vi "PID.vi"() -> ()   [LabVIEW 2016]
uses:
  <vilib>/addons/control/pid/autopid.llb/PID autotuning parameters (adv).ctl
  <vilib>/Analysis/baseanly.llb/Mean (DBL).vi
  <userlib>/Fluigent/Fluigent MFCS/FluigentMFCS_Full.llb/MFCS_EZ Detect.vi
  <userlib>/Fluigent/Fluigent MFCS/FluigentMFCS_Full.llb/MFCS_EZ Initialization.vi
  <userlib>/Fluigent/Fluigent MFCS/FluigentMFCS_Full.llb/MFCS_EZ Read All Channels Pressure.vi
  <userlib>/Fluigent/Fluigent MFCS/FluigentMFCS_Full.llb/MFCS_EZ Write Channel Pressure.vi
  <vilib>/addons/control/pid/NI_PID_autopid.lvlib
  <vilib>/Analysis/NI_AALBase.lvlib
  <vilib>/addons/control/pid/autopid.llb/PID Autotuning Design (Auto).vi
panel:
  in  "Set PID Gains":T1={"proportional gain (Kc)"=1.0, "integral time (Ti, min)"=0.01, "derivative time (Td, min)"=0.0} {"derivative time (Td, min)" format="%#.6g"; "integral time (Ti, min)" format="%#.6g"; "proportional gain (Kc)" format="%#.6g"}
  in  "Fwater":dbl
  in  "Channels":enum16{"1", "2", "3", "4", "5", "6", "7", "8"}[](array[ring])=[enum."4", enum."5"]
  in  "Boards":enum16{"A", "B", "C"}[](array[ring])=[enum."A", enum."A"]
  out "error out":errorcluster
  out "dt":dbl
  in  "Filter Size":i32=5
  out "Filtered Flow":dbl format="%0.2f"
  out "Feedback Signal":dbl[](graph)
  out "Current F1":dbl
  out "tuning completed?":bool
  in  "Accept new parameters":bool
  out "tuned PID gains":T1={"proportional gain (Kc)"=1.0, "integral time (Ti, min)"=0.01, "derivative time (Td, min)"=0.0} {"derivative time (Td, min)" format="%#.6g"; "integral time (Ti, min)" format="%#.6g"; "proportional gain (Kc)" format="%#.6g"}
  in  "auto? (F)":bool
  in  "autotuning parameters":T2={"technique"=1, "type of controller"=1, "control specification"=0, "amplitude"=10.0} {"amplitude" format="%.2f"; "control specification" items=["normal", "fast", "slow"]; "type of controller" items=["P", "PI", "PID"]; "technique" items=["Step Open Loop", "Step Closed Loop", "Relay", "PID Relay"]}
  in  "reinitialize? (F)":bool
  in  "autotune? (F)":bool
  in  "Manual Pressure Set":dbl
  in  "Feedback on":bool
  out "Flow Rate":dbl[](graph)
  out "Pressure":dbl[](graph)
  in  "stop":bool
  out "Pressure":dbl
  out "Feedback Signal":dbl format="%.2f"
  in  "Flow Setpoint":dbl format="%.2f"
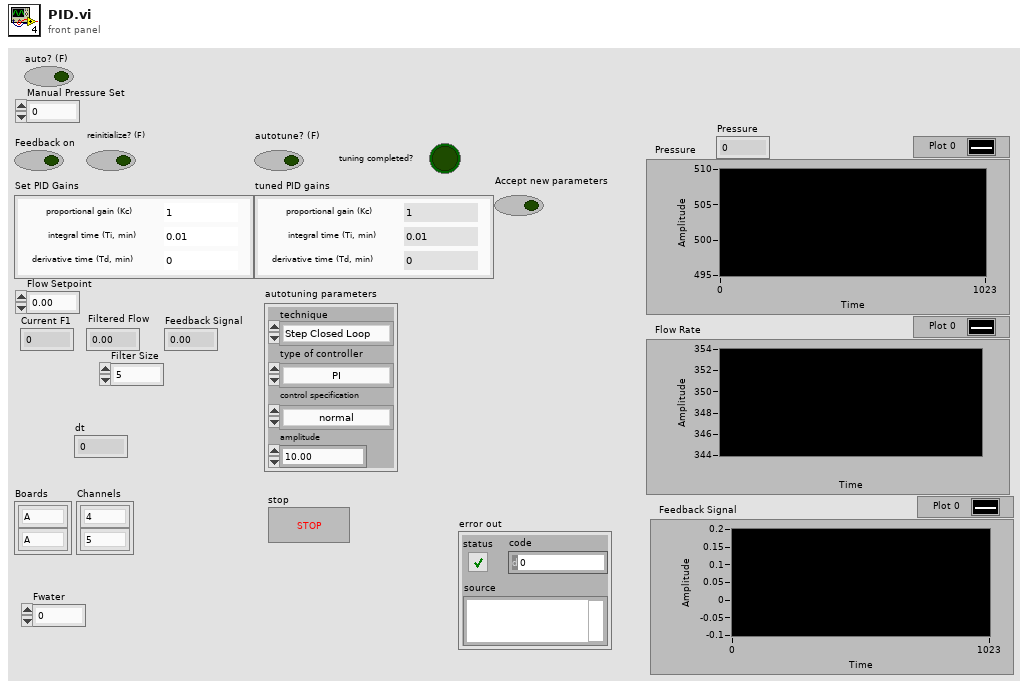
[diagram p1: front panel]
types:
  T1 = cluster{"proportional gain (Kc)":dbl, "integral time (Ti, min)":dbl, "derivative time (Td, min)":dbl}
  T2 = typedef "NI_PID_autopid.lvlib/PID autotuning parameters (adv).ctl" = cluster{"technique":u16, "type of controller":u16, "control specification":u16, "amplitude":dbl}
  T3 = typedef "_EZmfcsSN.ctl" = u16
  T4 = typedef "_frpRefNum" = refnum<k1>
  T5 = typedef "_EZmfcsRefNum.ctl" = refnum<k1>
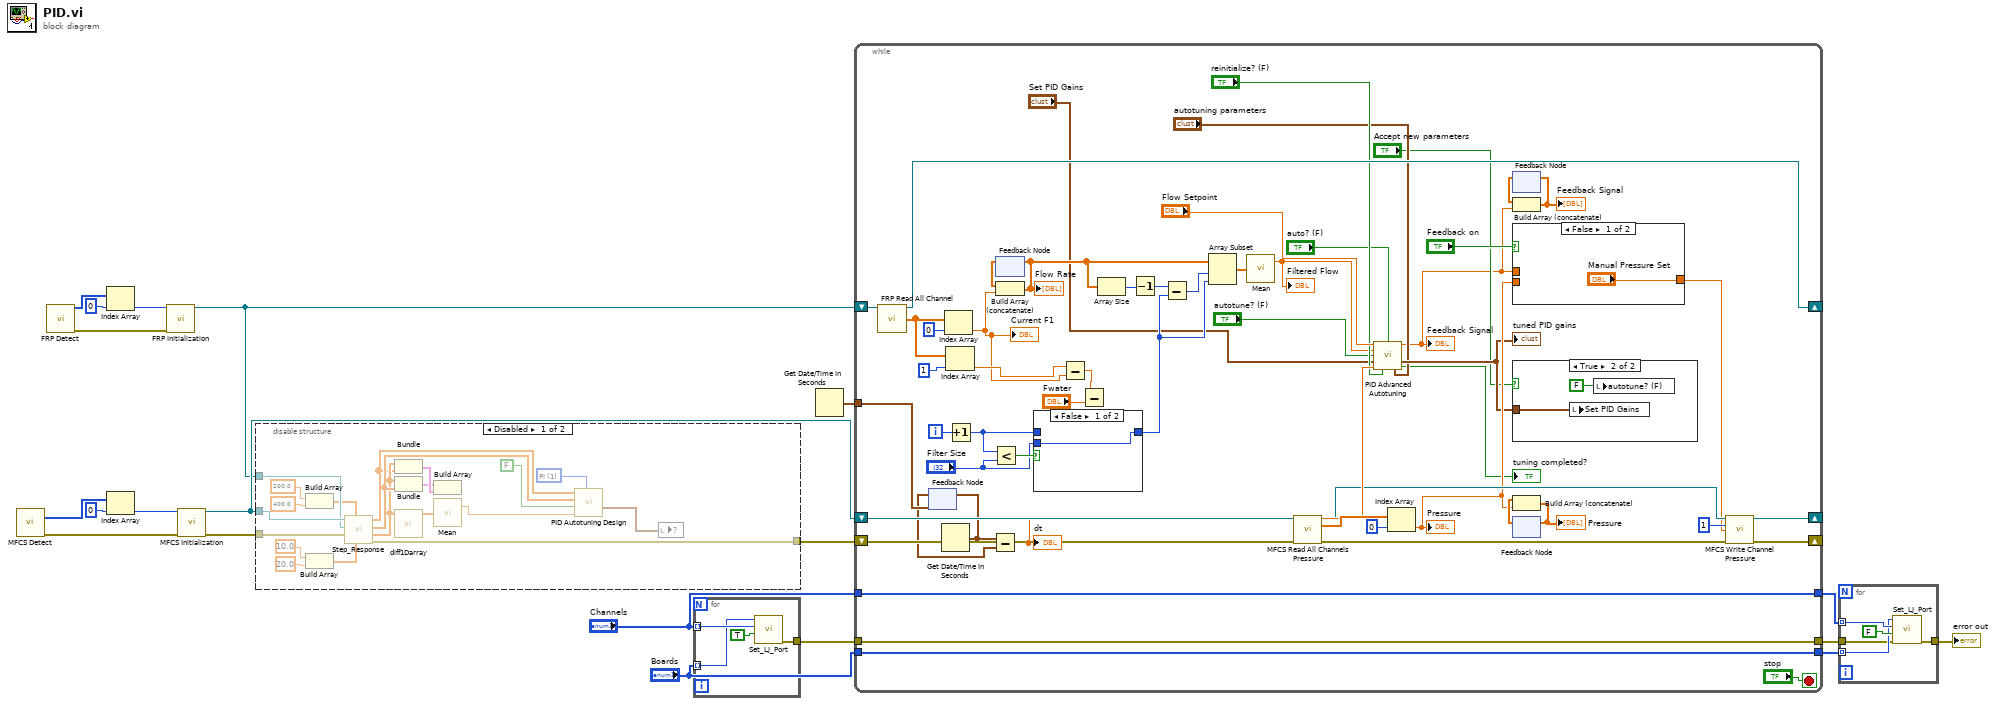
[diagram p0: block diagram]
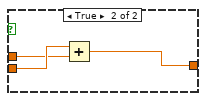
[diagram p5: hidden frame]
diagram:
  n1 = call-poly <userlib>:"MFCS Detect.vi"() -> ("[SN MFCS_EZ]"=w20:T3[], "error out"=w18:errorcluster)  [unwired: 14 in]
  n2 = call <userlib>:"FRP Detect.vi"() -> ("FLOWBOARD List"=w17:u16[], "error out"=w14:errorcluster)  [unwired: 14 in]
  n3 = Index Array(array=w17, index=0) -> (element=w13:u16)
  n4 = Index Array(array=w20, index=0) -> (element=w19:T3)
  n5 = call <userlib>:"FRP Initialization.vi"("Serial Number"=w13, "error in (no error)"=w14) -> ("FRP out"=w11:T4)  [unwired: 11 in, 2 out]
  n6 = call-poly <userlib>:"MFCS Initialization.vi"("SN MFCS_EZ"=w19, "error in (no error)"=w18) -> ("MFCS_EZ"=w12:T5, "error out"=w9:errorcluster)  [unwired: 11 in, 1 out]
  n7 = disable-structure shown="Disabled" {
    disable-tunnel: w12 -> [w42 _]
    disable-tunnel: w11 -> [w41 _]
    disable-tunnel: [w33 w43] -> w10
    disable-tunnel: w9 -> [w32 w43]
    frame Disabled {
      w37 = u16 1 items=["P", "PI", "PID"] ("Type of Controller")
      n8 = Build Array(200.0 ("element"), 400.0 ("element")) -> (w25:dbl[])
      n9 = Build Array(10.0 ("element"), 20.0 ("element")) -> (w26:dbl[])
      n10 = call "Step_Response.vi"("Times"=w26, "Pressure Sets"=w25, "MFCS Error"=w32, "FRP Handle"=w41, "MFCS Handle"=w42) -> ("error out"=w33:errorcluster, "T"=w24:dbl[], "Flow Rate"=w27:dbl[], "Pressure Setpoint"=w23:dbl[])  [unwired: 3 in]
      n11 = Bundle("T"=w24, "Pressure Setpoint"=w23) -> (w22:cluster{"T":dbl[], "Pressure Setpoint":dbl[]})  [unwired: 1 in]
      n12 = Bundle("T"=w24, "Flow Rate"=w27) -> (w21:cluster{"T":dbl[], "Flow Rate":dbl[]})  [unwired: 1 in]
      n13 = call "diff1Darray.vi"("Input"=w24) -> ("Diff"=w39:dbl[])  [unwired: 10 in]
      n14 = Build Array(w21, w22) -> ()  [unwired: 1 out]
      n15 = call-poly <vilib>:"Mean.vi"("X"=w39) -> ("mean"=w38:dbl)  [unwired: 1 out]
      n16 = call-poly <vilib>:"PID Autotuning Design.vi"("Type of Controller"=w37, "dt (s)"=w38, "closed-loop?"=FALSE, "Response signal"=w27, "Stimulus signal"=w23) -> ("PID gains"=w36:T1, "response operating point"=w34:dbl, "stimulus operating point"=w35:dbl)  [unwired: 3 in, 1 out]
      n17 = local write item#-1(w36) -> ()
    }
    frame Enabled {
    }
  }
  n18 = for {
    tunnel: "Channels" -> [w47] mode=indexing
    tunnel: "Boards" -> [w46] mode=indexing
    tunnel: [w44] -> w7
    n19 = call "Set_LJ_Port.vi"("State"=TRUE, "Channel"=w47, "Flowboard"=w46) -> ("error out"=w44:errorcluster)  [unwired: 8 in]
  }
  n20 = Get Date/Time In Seconds() -> (seconds since 1Jan1904=w8:timestamp)
  n21 = while {
    shift-right: [w91] -> _
    shift-left: w10 -> [w101]
    shift-right: [w90] -> _
    shift-left: w12 -> [w102]
    shift-right: [w97] -> _
    shift-left: w11 -> [w98]
    tunnel: [w55] -> w2
    tunnel: w7 -> [w55]
    tunnel: w8 -> [w81]
    tunnel: "Boards" -> [w56]
    tunnel: "Channels" -> [w57]
    tunnel: [w57] -> w4
    tunnel: [w56] -> w3
    i -> [w68]
    stop <- "stop" stop-if-true
    n22 = call <userlib>:"FRP Read All Channel.vi"("FRP"=w98) -> ("FRP out"=w97:T4, "All Flow-Rates"=w53:dbl[])  [unwired: 12 in, 1 out]
    n23 = feedback #1(w81) -> (w79:timestamp)
    n24 = Get Date/Time In Seconds() -> (seconds since 1Jan1904=w80:timestamp)
    n25 = feedback-in #1(w80) -> ()
    n26 = Index Array(array=w53, index=0) -> (element=w51:dbl)
    "Current F1" <- w51
    n27 = Index Array(array=w53, index=1) -> (element=w52:dbl)
    n28 = Increment(x=w68) -> (x+1=w66:i32)
    n29 = Subtract(x=w80, y=w79) -> (x-y=w94:dbl)
    "dt" <- w94
    n30 = Less?(x=w66, y="Filter Size") -> (x < y?=w67:bool)
    n31 = feedback #2() -> (w85:dbl[])  [unwired: 1 in]
    n32 = Build Array (concatenate)(w85, w51) -> (w61:dbl[])
    "Flow Rate" <- w61
    n33 = feedback-in #2(w61) -> ()
    n34 = case shown="False" w67 {
      tunnel: w66 -> [_ w104]
      tunnel: [w103 w104] -> w63
      tunnel: "Filter Size" -> [w103 _]
      frame False {
      }
      frame True {
      }
    }
    n35 = Subtract(x=w52, y=w51) -> (x-y=w50:dbl)
    n36 = Subtract(x=w50, y="Fwater") -> ()  [unwired: 1 out]
    n37 = Array Size(array=w61) -> (size(s)=w64:i32)
    n38 = Decrement(x=w64) -> (x-1=w62:i32)
    n39 = Subtract(x=w62, y=w63) -> (x-y=w60:i32)
    n40 = Array Subset(array=w61, index=w60, length=w63) -> (w59:dbl[])
    n41 = call-poly <vilib>:"Mean.vi"("X"=w59) -> ("mean"=w58:dbl)  [unwired: 1 out]
    "Filtered Flow" <- w58
    n42 = call-poly <userlib>:"MFCS Read All Channels Pressure.vi"("MFCS_EZ"=w102, "error in (no error)"=w101) -> ("MFCS_EZ out"=w93:T5, "All Channels Pressure"=w96:dbl[], "error out"=w92:errorcluster)  [unwired: 11 in]
    n43 = call <vilib>:"PID Advanced Autotuning.vi"("setpoint"="Flow Setpoint", "auto? (F)"="auto? (F)", "process variable"=w58, "autotune? (F)"="autotune? (F)", "PID gains"="Set PID Gains", "dt (s)"=w94, "reinitialize? (F)"="reinitialize? (F)", "autotuning parameters"="autotuning parameters") -> ("output"=w71:dbl, "tuned PID gains"=w77:T1, "tuning completed?"=→"tuning completed?":bool)  [unwired: 5 in]
    "Feedback Signal" <- w71
    "tuned PID gains" <- w77
    n44 = Index Array(array=w96, index=0) -> (element=w84:dbl)
    "Pressure" <- w84
    n45 = feedback #3() -> (w70:dbl[])  [unwired: 1 in]
    n46 = Build Array (concatenate)(w70, w71) -> (w69:dbl[])
    "Feedback Signal" <- w69
    n47 = feedback-in #3(w69) -> ()
    n48 = case shown="False" "Feedback on" {
      tunnel: w84 -> [_ w110]
      tunnel: w71 -> [_ w109]
      tunnel: ["Manual Pressure Set" w108] -> w83
      frame False {
      }
      frame True {
        n49 = Add(x=w110, y=w109) -> (x+y=w108:dbl)
      }
    }
    n50 = case shown="True" "Accept new parameters" {
      tunnel: w77 -> [_ w106]
      frame False {
      }
      frame True {
        n51 = local write "Set PID Gains"(w106) -> ()
        n52 = local write "autotune? (F)"(FALSE ("autotune? (F)")) -> ()
      }
    }
    n53 = feedback #4() -> (w87:dbl[])  [unwired: 1 in]
    n54 = Build Array (concatenate)(w87, w84) -> (w86:dbl[])
    "Pressure" <- w86
    n55 = feedback-in #4(w86) -> ()
    n56 = call-poly <userlib>:"MFCS Write Channel Pressure.vi"("MFCS_EZ"=w93, "Channel Number (default=1)"=u8 1, "Pressure (mBar)"=w83, "error in (no error)"=w92) -> ("MFCS_EZ out"=w90:T5, "error out"=w91:errorcluster)  [unwired: 10 in]
  }
  n57 = for {
    tunnel: w4 -> [w115] mode=indexing
    tunnel: [w113] -> w1
    tunnel: w3 -> [w112] mode=indexing
    tunnel: w2 -> [w111]
    n58 = call "Set_LJ_Port.vi"("error in"=w111, "State"=FALSE, "Channel"=w115, "Flowboard"=w112) -> ("error out"=w113:errorcluster)  [unwired: 7 in]
  }
  "error out" <- w1
